vi "CalcFrequency.vi"(8 "BScanPerCScan":dbl, 9 "AScanPerBScan":dbl, 11 "AScanFrequency":dbl) -> (0 "SlowPeriod":dbl, 1 "FastPeriod":dbl, 2 "SlowFrequency":dbl, 3 "FastFrequency":dbl)   [LabVIEW 2019]
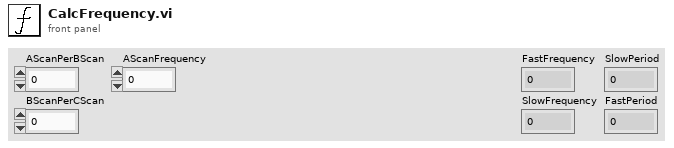
[diagram p1: front panel]
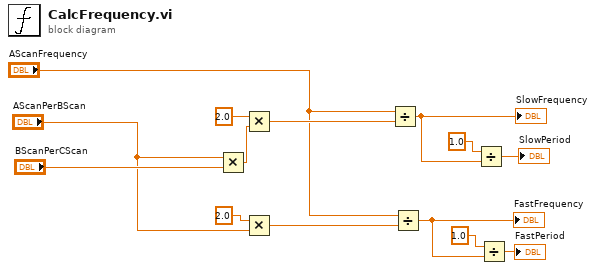
[diagram p0: block diagram]
diagram:
  n1 = Multiply(x="AScanPerBScan", y="BScanPerCScan") -> (x*y=w13:dbl)
  n2 = Multiply(x=2.0, y=w13) -> (x*y=w14:dbl)
  n3 = Multiply(x=2.0, y="AScanPerBScan") -> (x*y=w10:dbl)
  n4 = Divide(x="AScanFrequency", y=w14) -> (x/y=w5:dbl)
  "SlowFrequency" <- w5
  n5 = Divide(x="AScanFrequency", y=w10) -> (x/y=w2:dbl)
  "FastFrequency" <- w2
  n6 = Divide(x=1.0, y=w5) -> (x/y=→"SlowPeriod":dbl)
  n7 = Divide(x=1.0, y=w2) -> (x/y=→"FastPeriod":dbl)
